vi "Comb.vi"(10 "sample":bool=TRUE, 11 "data in":bool[](array[boolean])) -> (0 "ready for input":bool, 2 "output valid":bool, 3 "data out":bool[](array[boolean]))   [LabVIEW 2011]
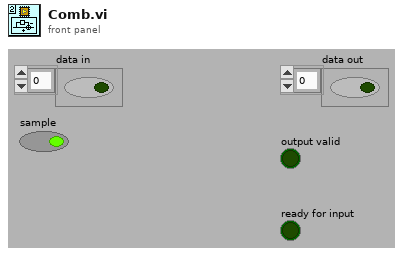
[diagram p1: front panel]
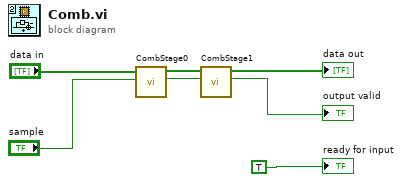
[diagram p0: block diagram]
diagram:
  n1 = call "CombStage0.vi"("input valid"="sample", "data in"="data in") -> ("output valid"=w3:bool, "data out"=w4:bool[])  [unwired: 8 in]
  n2 = call "CombStage1.vi"("input valid"=w3, "data in"=w4) -> ("output valid"=→"output valid":bool, "data out"=→"data out":bool[])  [unwired: 8 in]
  "ready for input" <- TRUE
